vi "Call_IDL.vi"(7 "Arguments":string[](array[string]), 8 "error in (no error)":errorcluster, 11 "IDL function":string) -> (0 "error out":errorcluster, 2 "Unedited Return String":string, 3 "Return Values":string[](array[string]), 4 "standard error":string, 5 "standard output":string)   [LabVIEW 2013]
uses:
  <userlib>/_OpenG.lib/string/string.llb/Trim Whitespace (String)__ogtk.vi
  <userlib>/_OpenG.lib/string/string.llb/Trim Whitespace (String Array)__ogtk.vi
  <userlib>/_OpenG.lib/array/array.llb/Conditional Auto-Indexing Tunnel (String)__ogtk.vi
panel:
  out "IDL Command Line":string="\"C:\\Program Files\\Exelis\\IDL82\\bin\\bin.x86_64\\idl.exe\" -e  \"multiply, '2', '3'\""
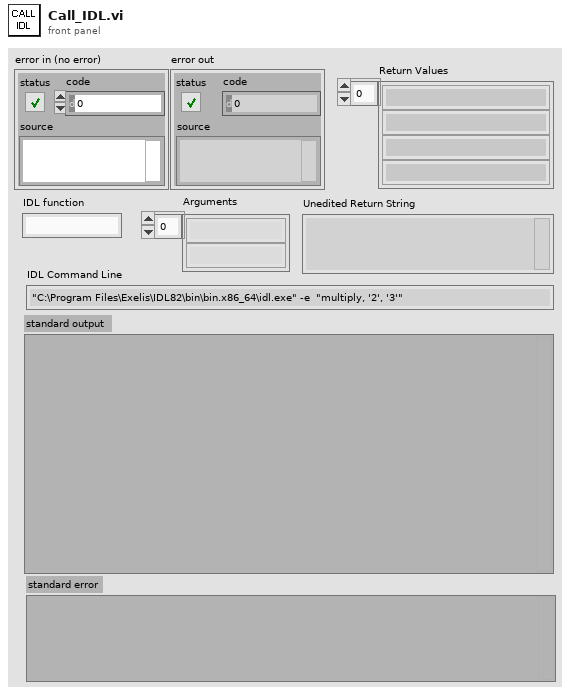
[diagram p1: front panel]
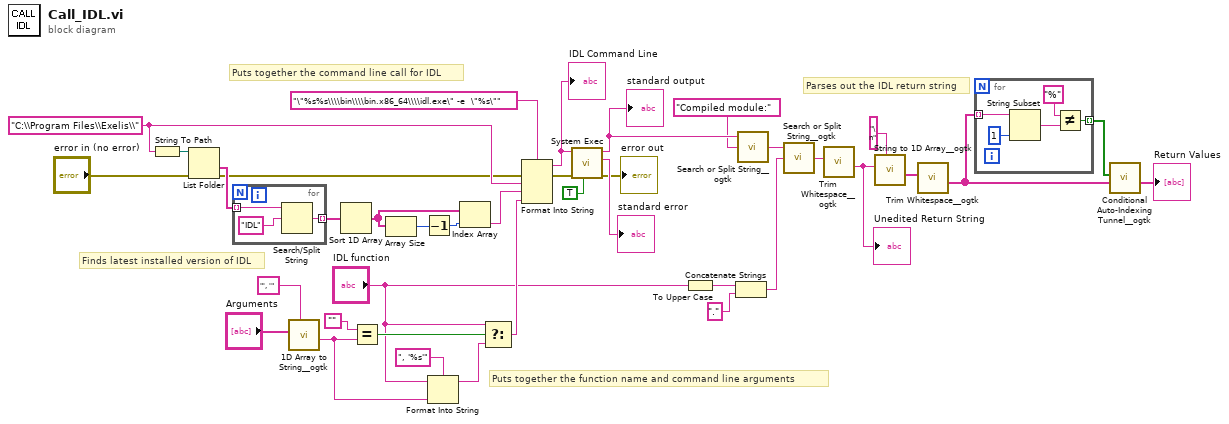
[diagram p0: block diagram]
diagram:
  w37 = "C:\\Program Files\\Exelis\\"
  # "Parses out the IDL return string"
  # "Puts together the command line call for IDL"
  # "Puts together the function name and command line arguments"
  # "Finds latest installed version of IDL"
  n1 = String To Path(string=w37) -> (path=w31:path)
  n2 = List Folder(path=w31, error in="error in (no error)") -> (folder names=w32:string[], error out=w30:errorcluster)  [unwired: 2 in, 2 out]
  n3 = for {
    tunnel: w32 -> [w40] mode=indexing
    tunnel: [w39] -> w34 mode=indexing
    n4 = Search/Split String(string=w40, search string/char (-)="IDL" ("Element Data")) -> (match + rest of string=w39:string)  [unwired: 1 in, 2 out]
  }
  n5 = call <userlib>:"1D Array to String__ogtk.vi"("delimiter (Tab)"="', '", "Array of Strings"="Arguments") -> ("delimited string"=w21:string)  [unwired: 9 in]
  n6 = Sort 1D Array(array=w34) -> (sorted array=w33:string[])
  n7 = Equal?(x="", y=w21) -> (x = y?=w23:bool)
  n8 = Array Size(array=w33) -> (size(s)=w35:i32)
  n9 = Decrement(x=w35) -> (x-1=w36:i32)
  n10 = Format Into String(format string=", '%s'", initial string="IDL function", w21) -> (resulting string=w20:string)  [unwired: 1 in, 1 out]
  n11 = Index Array(array=w33, index=w36) -> (element=w38:string)
  n12 = Select(t="IDL function", s=w23, f=w20) -> (s? t:f=w19:string)
  n13 = Format Into String(format string="\"%s%s\\\\bin\\\\bin.x86_64\\\\idl.exe\" -e  \"%s\"", error in=w30, w37, w38, w19) -> (resulting string=w4:string, error out=w18:errorcluster)  [unwired: 1 in]
  "IDL Command Line" <- w4
  n14 = call <vilib>:"System Exec.vi"("run minimized? (F)"=TRUE, "error in (no error)"=w18, "command line"=w4) -> ("error out"=→"error out":errorcluster, "standard error"=→"standard error":string, "standard output"=w15:string)  [unwired: 5 in, 1 out]
  "standard output" <- w15
  n15 = To Upper Case(1:"IDL function") -> (0:w8:string)
  n16 = Concatenate Strings(w8, "." ("search string/char (-)")) -> (w7:string)
  n17 = call <userlib>:"Search or Split String__ogtk.vi"("search string/char (-)"="Compiled module:", "string"=w15) -> ("substring after match"=w12:string)  [unwired: 1 in, 2 out]
  n18 = call <userlib>:"Search or Split String__ogtk.vi"("search string/char (-)"=w7, "string"=w12) -> ("substring after match"=w11:string)  [unwired: 1 in, 2 out]
  n19 = call-poly <userlib>:"Trim Whitespace__ogtk.vi"("String in"=w11) -> ("String out"=w9:string)  [unwired: 6 in]
  "Unedited Return String" <- w9
  n20 = call <userlib>:"String to 1D Array__ogtk.vi"("delimiter (Tab)"="\n", "string"=w9) -> ("Array of Strings"=w10:string[])  [unwired: 9 in]
  n21 = call-poly <userlib>:"Trim Whitespace__ogtk.vi"("String in"=w10) -> ("String out"=w2:string[])  [unwired: 6 in]
  n22 = for {
    tunnel: w2 -> [w46] mode=indexing
    tunnel: [w42] -> w1 mode=indexing
    n23 = String Subset(string=w46, length (rest)=1 ("length (rest)")) -> (substring=w44:string)  [unwired: 1 in]
    n24 = Not Equal?(x="%", y=w44) -> (x != y?=w42:bool)
  }
  n25 = call-poly <userlib>:"Conditional Auto-Indexing Tunnel__ogtk.vi"("Array in"=w2, "Elements to keep"=w1) -> ("Filtered Array out"=→"Return Values":string[])  [unwired: 5 in]
